vi "JSON to TOML.vi"(10 "JSON Value":T1) -> (2 "Value":T2)   [LabVIEW 2017]
uses:
  <vilib>/Erdos Miller/LV-JSON/JSON Value.ctl
  src/lib/TOML Value.ctl
  src/lib/TOML.lvlib
  <vilib>/Erdos Miller/LV-JSON/JSON Name-Value Pair.ctl
  src/lib/TOML Key-Value Pair.ctl
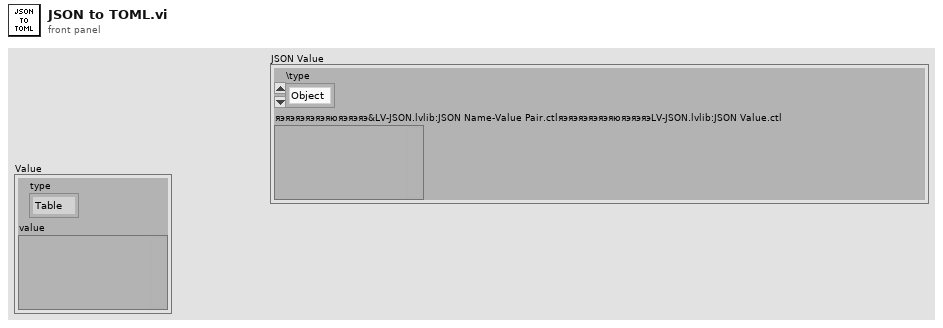
[diagram p1: front panel]
types:
  T1 = typedef "LV-JSON.lvlib/JSON Value.ctl" = cluster{"\\type":enum16{"Object", "Array", "String", "Number", "Boolean", "Null"}, "яэяэяэяэяэяюяэяэяэ&LV-JSON.lvlib:JSON Name-Value Pair.ctlяэяэяэяэяэяюяэяэяэLV-JSON.lvlib:JSON Value.ctl":variant}
  T2 = typedef "TOML.lvlib/TOML Value.ctl" = cluster{"type":enum16{"Table", "Array", "String", "Integer", "Float", "Boolean", "Offset Date-Time", "Local Date-Time", "Local Date", "Local Time"}, "value":variant}
  T3 = enum16{"Object", "Array", "String", "Number", "Boolean", "Null"}
  T4 = cluster{"Key":string, "\\type":enum16{"Object", "Array", "String", "Number", "Boolean", "Null"}, "Key":string}
  T5 = typedef "LV-JSON.lvlib/JSON Name-Value Pair.ctl" = cluster{"Name":string, "Value":T1}
  T6 = enum16{"Table", "Array", "String", "Integer", "Float", "Boolean", "Offset Date-Time", "Local Date-Time", "Local Date", "Local Time"}
  T7 = typedef "TOML.lvlib/TOML Key-Value Pair.ctl" = cluster{"Key":string, "Value":T2}
  T8 = cluster{"Name":string, "\\type":enum16{"Object", "Array", "String", "Number", "Boolean", "Null"}, "Name":string}
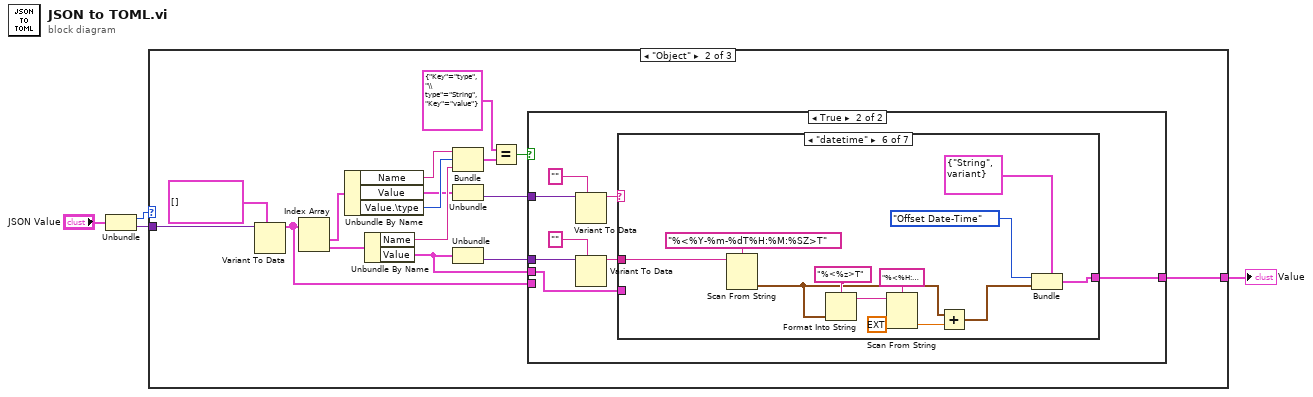
[diagram p0: block diagram]
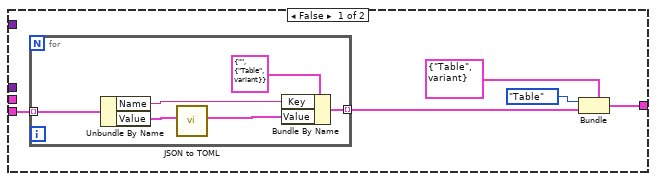
[diagram p3: hidden frame]
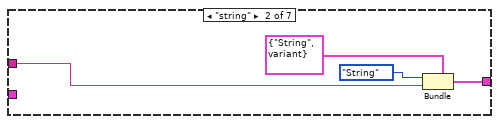
[diagram p5: hidden frame]
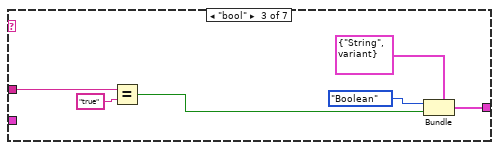
[diagram p6: hidden frame]
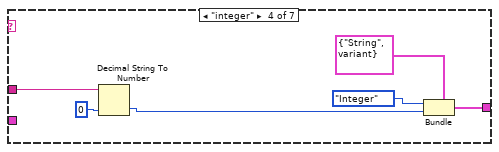
[diagram p7: hidden frame]
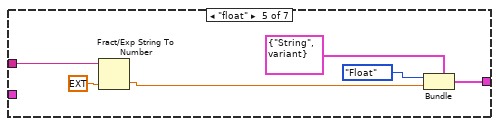
[diagram p8: hidden frame]
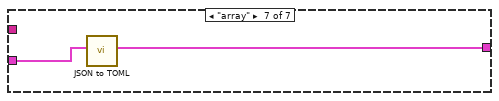
[diagram p9: hidden frame]
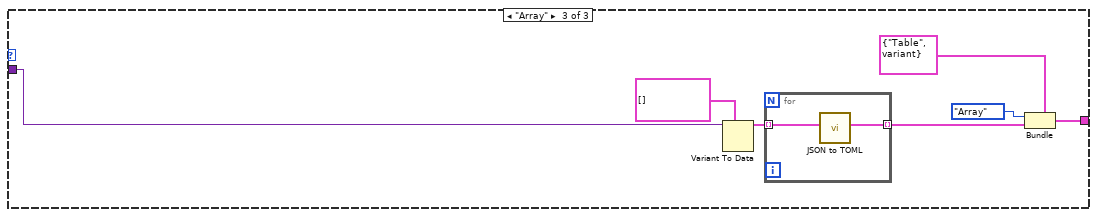
[diagram p10: hidden frame]
diagram:
  n1 = Unbundle("JSON Value") -> ("\\type"=w3:T3, "яэяэяэяэяэяюяэяэяэ&LV-JSON.lvlib:JSON Name-Value Pair.ctlяэяэяэяэяэяюяэяэяэLV-JSON.lvlib:JSON Value.ctl"=w4:variant)
  n2 = case shown="\"Object\"" w3 {
    tunnel: w4 -> [_ w20 w82]
    tunnel: [_ w18 w78] -> w1
    frame Default {
    }
    frame "Object" {
      n3 = Variant To Data(type=T5[] [], Variant=w20) -> (data=w17:T5[])  [unwired: 1 in, 1 out]
      n4 = Index Array(array=w17) -> (element #1=w16:T5, element #2=w15:T5)  [unwired: 2 in]
      n5 = Unbundle By Name(w16) -> ("Name"=w14:string, "Value"=w8:T1, "Value.\\type"=w13:T3)
      n6 = Unbundle By Name(w15) -> ("Name"=w12:string, "Value"=w5:T1)
      n7 = Bundle("Name"=w14, "\\type"=w13, "Name"=w12) -> (w11:T8)  [unwired: 1 in]
      n8 = Unbundle(w8) -> ("яэяэяэяэяэяюяэяэяэ&LV-JSON.lvlib:JSON Name-Value Pair.ctlяэяэяэяэяэяюяэяэяэLV-JSON.lvlib:JSON Value.ctl"=w7:variant)  [unwired: 1 out]
      n9 = Unbundle(w5) -> ("яэяэяэяэяэяюяэяэяэ&LV-JSON.lvlib:JSON Name-Value Pair.ctlяэяэяэяэяэяюяэяэяэLV-JSON.lvlib:JSON Value.ctl"=w6:variant)  [unwired: 1 out]
      n10 = Equal?(x=T4 {"Key"="type", "\\type"=enum."String", "Key"="value"}, y=w11) -> (x = y?=w9:bool)
      n11 = case shown="True" w9 {
        tunnel: [w25 w33] -> w18
        tunnel: w17 -> [w21 _]
        tunnel: w7 -> [_ w39]
        tunnel: w6 -> [_ w38]
        tunnel: w5 -> [_ w32]
        frame False {
          n12 = for {
            tunnel: w21 -> [w31] mode=indexing
            tunnel: [w27] -> w24 mode=indexing
            n13 = Unbundle By Name(w31) -> ("Name"=w29:string, "Value"=w30:T1)
            n14 = call "JSON to TOML.vi"("JSON Value"=w30) -> ("Value"=w28:T2)  [unwired: 10 in]
            n15 = Bundle By Name(cluster=T7 {"Key"="", "Value"={"type"=enum."Table", "value"=variant}} ("Key-Value Pair"), "Key"=w29, "Value"=w28) -> (w27:T7)
          }
          n16 = Bundle(cluster=T2 {"type"=enum."Table", "value"=variant} ("Value"), "type"=T6."Table" ("\\type"), "value"=w24) -> (w25:T2)
        }
        frame True {
          n17 = Variant To Data(type="", Variant=w39) -> (data=w35:string)  [unwired: 1 in, 1 out]
          n18 = Variant To Data(type="", Variant=w38) -> (data=w34:string)  [unwired: 1 in, 1 out]
          n19 = case shown="\"datetime\"" w35 {
            tunnel: w34 -> [_ w41 w46 w52 w58 w69 _]
            tunnel: [_ w40 w47 w53 w59 w71 w74] -> w33
            tunnel: w32 -> [_ _ _ _ _ _ w75]
            frame Default {
            }
            frame "string" {
              n20 = Bundle(cluster=T2 {"type"=enum."String", "value"=variant} ("Value"), "type"=T6."String" ("\\type"), "value"=w41) -> (w40:T2)
            }
            frame "bool" {
              n21 = Equal?(x=w46, y="true") -> (x = y?=w44:bool)
              n22 = Bundle(cluster=T2 {"type"=enum."String", "value"=variant} ("Value"), "type"=T6."Boolean" ("\\type"), "value"=w44) -> (w47:T2)
            }
            frame "integer" {
              n23 = Decimal String To Number(string=w52, default (0L)=i64 0 ("default (0 I32)")) -> (number=w51:i64)  [unwired: 1 in, 1 out]
              n24 = Bundle(cluster=T2 {"type"=enum."String", "value"=variant} ("Value"), "type"=T6."Integer" ("\\type"), "value"=w51) -> (w53:T2)
            }
            frame "float" {
              n25 = Fract/Exp String To Number(string=w58, default (0 dbl)=ext 0.0 ("default (0 I32)")) -> (number=w57:ext)  [unwired: 2 in, 1 out]
              n26 = Bundle(cluster=T2 {"type"=enum."String", "value"=variant} ("Value"), "type"=T6."Float" ("\\type"), "value"=w57) -> (w59:T2)
            }
            frame "datetime" {
              n27 = Scan From String(format string="%<%Y-%m-%dT%H:%M:%SZ>T", input string=w69) -> (output 1=w63:timestamp)  [unwired: 3 in, 3 out]
              n28 = Format Into String(format string="%<%z>T", w63) -> (resulting string=w66:string)  [unwired: 2 in, 1 out]
              n29 = Scan From String(format string="%<%H:%M:%S>t", input string=w66, default 1=ext 0.0 ("default value 1")) -> (output 1=w64:ext)  [unwired: 2 in, 3 out]
              n30 = Add(x=w63, y=w64) -> (x+y=w62:timestamp)
              n31 = Bundle(cluster=T2 {"type"=enum."String", "value"=variant} ("Value"), "type"=T6."Offset Date-Time" ("\\type"), "value"=w62) -> (w71:T2)
            }
            frame "array" {
              n32 = call "JSON to TOML.vi"("JSON Value"=w75) -> ("Value"=w74:T2)  [unwired: 10 in]
            }
          }
        }
      }
    }
    frame "Array" {
      n33 = Variant To Data(type=T1[] [], Variant=w82) -> (data=w80:T1[])  [unwired: 1 in, 1 out]
      n34 = for {
        tunnel: w80 -> [w84] mode=indexing
        tunnel: [w83] -> w79 mode=indexing
        n35 = call "JSON to TOML.vi"("JSON Value"=w84) -> ("Value"=w83:T2)  [unwired: 10 in]
      }
      n36 = Bundle(cluster=T2 {"type"=enum."Table", "value"=variant} ("Value"), "type"=T6."Array" ("\\type"), "value"=w79) -> (w78:T2)
    }
  }
  "Value" <- w1
